vi "关闭Excel.vi"(8 "错误输入（无错误）":errorcluster, 11 "文件路径":path=path "") -> (0 "错误输出":errorcluster)   [LabVIEW 2020, in "OperateExcel.lvlib"]
uses:
  OperateExcel.lvlib
  Globals.vi
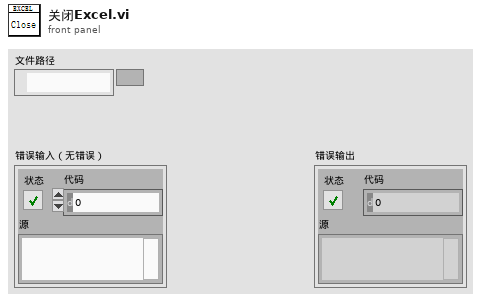
[diagram p1: front panel]
types:
  T1 = typedef "OperateExcel.lvlib/引用簇.ctl" = cluster{"Excel._Application":refnum<k7>, "Workbooks":refnum<k7>, "Open":refnum<k7>, "Worksheets":refnum<k7>, "sheetList":refnum<k7>[]}
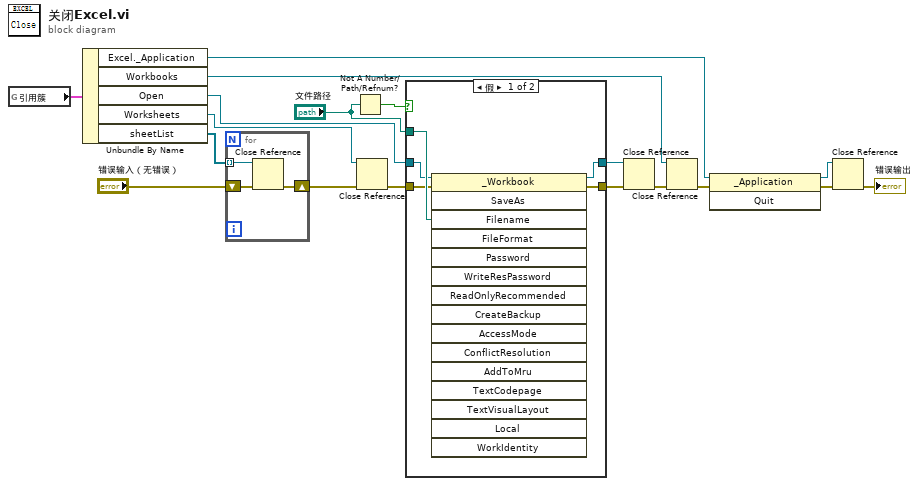
[diagram p0: block diagram]
diagram:
  n1 = global read "Globals.vi" "引用簇"() -> (w2:T1)
  n2 = Unbundle By Name(w2) -> ("Excel._Application"=w6:refnum<k7>, "Workbooks"=w7:refnum<k7>, "Open"=w12:refnum<k7>, "Worksheets"=w14:refnum<k7>, "sheetList"=w15:refnum<k7>[])
  n3 = for {
    tunnel: w15 -> [w21] mode=indexing
    shift-right: [w19] -> w13
    shift-left: "错误输入（无错误）" -> [w20]
    n4 = Close Reference(reference=w21, error in (no error)=w20) -> (error out=w19:errorcluster)
  }
  n5 = Not A Number/Path/Refnum?(number/path/refnum="文件路径") -> (NaN/Path/Refnum?=w1:bool)
  n6 = Close Reference(reference=w14, error in (no error)=w13) -> (error out=w11:errorcluster)
  n7 = case shown="假" w1 {
    tunnel: "文件路径" -> [w26 _]
    tunnel: w12 -> [w25 w28]
    tunnel: w11 -> [w24 w27]
    tunnel: [w23 w28] -> w10
    tunnel: [w22 w27] -> w9
    frame False {
      n8 = invoke class="_Workbook" method="SaveAs"(reference=w25, error in=w24, "Filename"=w26) -> (reference out=w23:refnum<k7>, error out=w22:errorcluster)  [unwired: 13 in, 14 out]
    }
    frame True {
    }
  }
  n9 = Close Reference(reference=w10, error in (no error)=w9) -> (error out=w8:errorcluster)
  n10 = Close Reference(reference=w7, error in (no error)=w8) -> (error out=w5:errorcluster)
  n11 = invoke class="_Application" method="Quit"(reference=w6, error in=w5) -> (reference out=w3:refnum<k7>, error out=w4:errorcluster)  [unwired: 1 in, 1 out]
  n12 = Close Reference(reference=w3, error in (no error)=w4) -> (error out=→"错误输出":errorcluster)
